vi "DecideWhenToShift.vi"(4 "Shifter State":bool, 5 "Wheel Velocity (rpm)":dbl, 6 "Time Below Speed (ms)":u32, 7 "Time Above Speed (ms)":u32, 8 "Switch to Low Gear (ft/s)":dbl, 9 "Switch to High Gear (ft/s)":dbl) -> (3 "Output":bool)   [LabVIEW 2019]
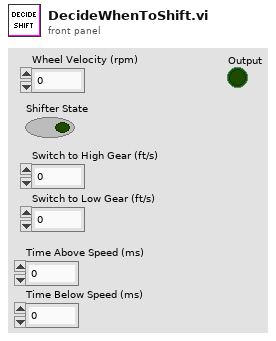
[diagram p1: front panel]
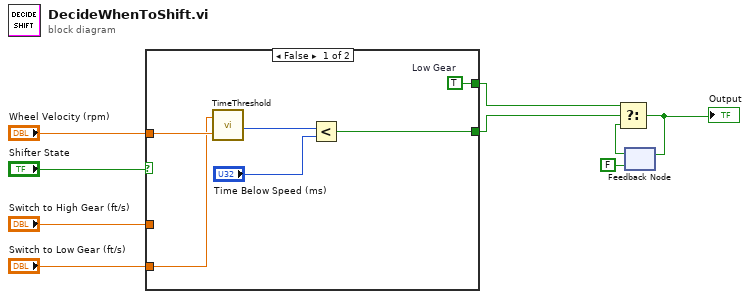
[diagram p0: block diagram]
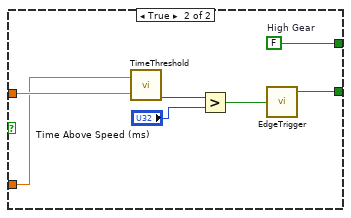
[diagram p2: hidden frame]
diagram:
  n1 = case shown="False" "Shifter State" {
    tunnel: "Wheel Velocity (rpm)" -> [w15 w22]
    tunnel: "Switch to High Gear (ft/s)" -> [_ w21]
    tunnel: "Switch to Low Gear (ft/s)" -> [w14 _]
    tunnel: [w11 w17] -> w5
    tunnel: [w10 w16] -> w4
    frame False {
      w10 = TRUE  # Low Gear
      n2 = call "TimeThreshold.vi"("Threshold"=w15, "Current Value"=w14) -> ("Time Below Threshold (ms)"=w13:u32)  [unwired: 1 out]
      n3 = Less?(x=w13, y="Time Below Speed (ms)") -> (x < y?=w11:bool)
    }
    frame True {
      w16 = FALSE  # High Gear
      n4 = call "TimeThreshold.vi"("Threshold"=w22, "Current Value"=w21) -> ("Time Above Threshold (ms)"=w20:u32)  [unwired: 1 out]
      n5 = Greater?(x=w20, y="Time Above Speed (ms)") -> (0:w18:bool)
      n6 = call "EdgeTrigger.vi"("Input Signal"=w18) -> ("Rising Edge Trigger"=w17:bool)  [unwired: 2 out]
    }
  }
  n7 = feedback #1(FALSE ("High Gear")) -> (w3:bool)
  n8 = Select(t=w4, s=w5, f=w3) -> (s? t:f=w1:bool)
  "Output" <- w1
  n9 = feedback-in #1(w1) -> ()
